vi "avg_of_num.vi"() -> ()   [LabVIEW 2026]
panel:
  out "(^_^)":dbl
  in  "b":dbl
  in  "a":dbl
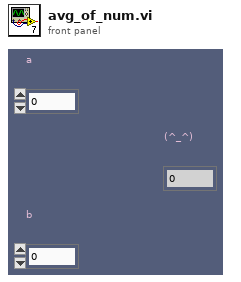
[diagram p1: front panel]
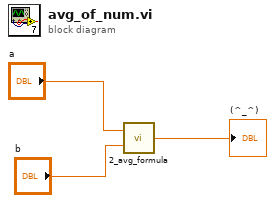
[diagram p0: block diagram]
diagram:
  n1 = call "2_avg_formula.vi"("B"="b", "A"="a") -> ("OP"=→"(^_^)":dbl)
